vi "gxml_RcrsvFlatten.vi"(5 "Encap'd by Array?":bool, 6 "HierarchyInfo":T1, 7 "FlattenedData":string, 8 "error in":errorcluster, 9 "offset (0)":i32, 10 "Variant":variant, 11 "XML String In":string) -> (0 "error out":errorcluster, 1 "offset out":i32, 3 "XML String Out":string)   [LabVIEW 2011, in "Third Party VIs.lvlib" / "GXML.lvlib"]
doc: "This recursive VI is the core engine responsible for converting the LabVIEW cluster into an XML string. \n\nThe VI identifies the top level datatype of the input variant and recursively calls itself when an encapsulaing datatype is found (ie cluster or array). When a fundamental item is found (integer, boolean, etc) it is converted to text and given tags with appropriate attributes and hierarchy."
uses:
  GXML.lvlib
  <vilib>/Utility/VariantDataType/VariantType.lvlib
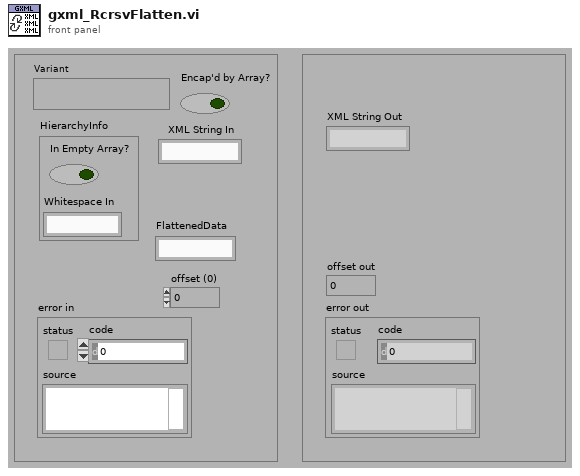
[diagram p1: front panel]
types:
  T1 = cluster{"In Empty Array?":bool, "Whitespace In":string}
  T2 = typedef "VariantType.lvlib/Type.ctl" = enum8{"Invalid Type", "Void", "I8", "I16", "I32", "I64", "U8", "U16", "U32", "U64", "Single Float", "Double Float", "Extended Float", "Single Complex", "Double Complex", "Extended Complex", "Enum U8", "Enum U16", "Enum U32", "Enum U64", "Single Float With Unit", "Double Float With Unit", "Extended Float With Unit", "Single Complex with Unit", "Double Complex with Unit", "Extended Complex with Unit", "Boolean", "String", "Path", "Picture", "Tag", "Array", "Cluster", "Variant", "LV Variant", "Waveform", "Timestamp", "Digital Waveform", "Digital Data", "ExpressData", "Refnum", "External Data", "VI", "Poly VI", "LabVIEW Class Instance", "Fixed Point"}
  T3 = cluster{"TypeAttr":string, "EnumSelAttr":string, "DataString":string}
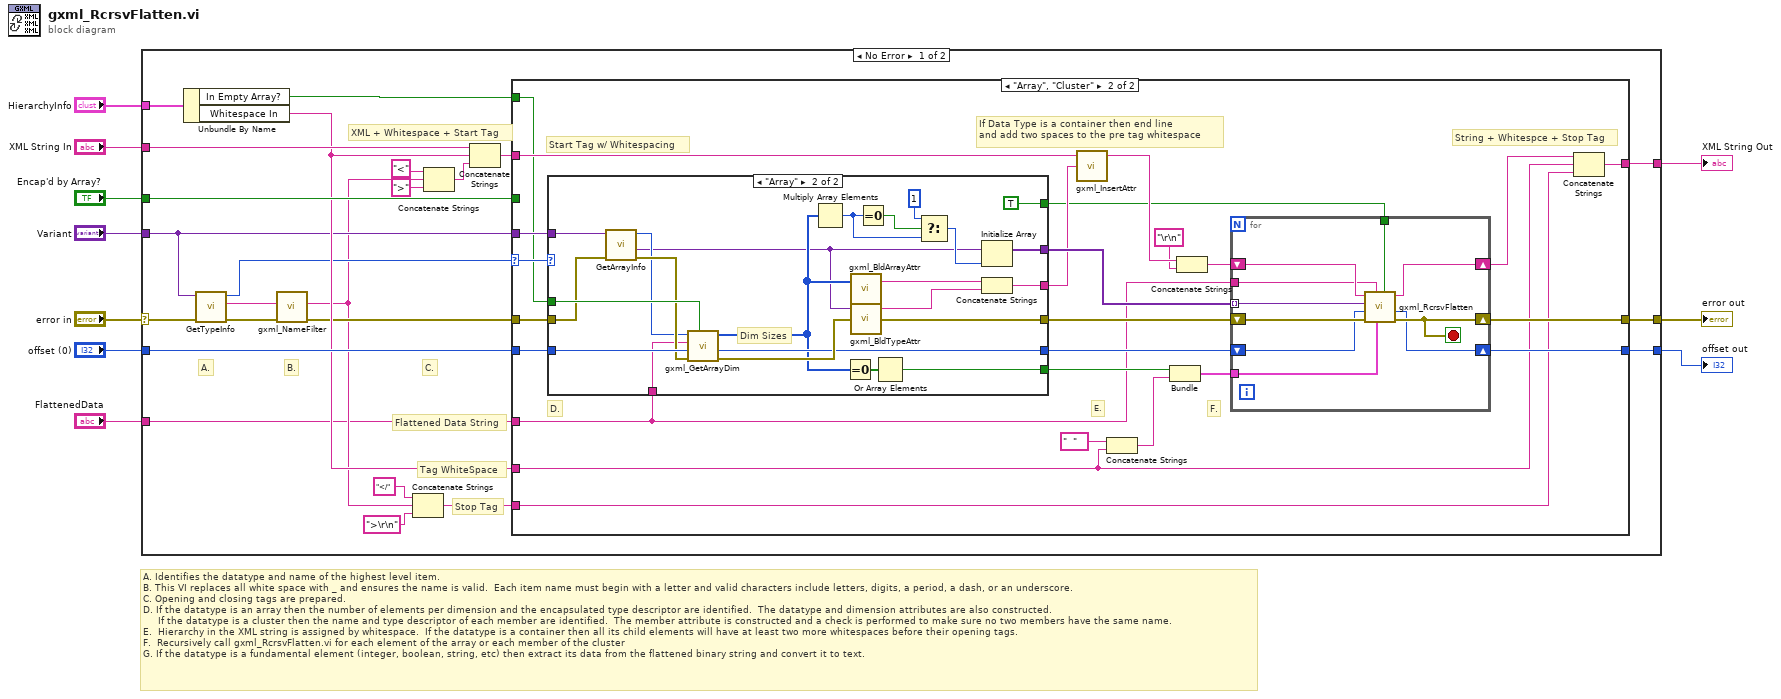
[diagram p0: block diagram]
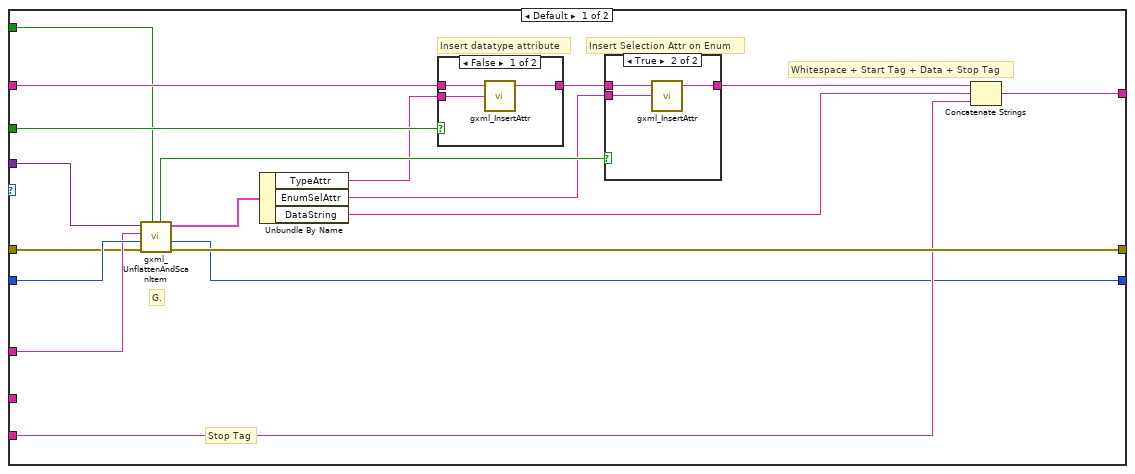
[diagram p2: hidden frame]
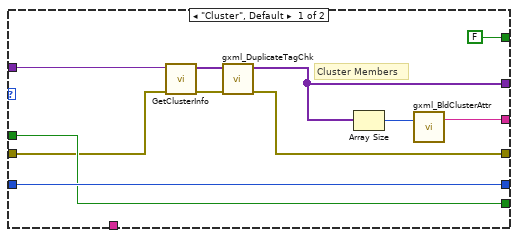
[diagram p5: hidden frame]
diagram:
  # "A. Identifies the datatype and name of the highest level item.\nB. This VI replaces all white space with _ and ensures the name is valid.  Each item name must begin with a letter and valid characters include letters, digits, a period, a dash, or an underscore.\nC. Opening and closing tags are prepared.\nD. If the datatype is an array then the number of elements per dimension and the encapsulated type descriptor are identified.  The datatype and dimension attributes are also constructed.\n     If the datatype is a cluster then the name and type descriptor of each member are identified.  The member attribute is constructed and a check is performed to make sure no two members have the same name.\nE.  Hierarchy in the XML string is assigned by whitespace.  If the datatype is a container then all its child elements will have at least two more whitespaces before their opening tags.\nF.  Recursively call gxml_RcrsvFlatten.vi for each element of the array or each member of the cluster\nG. If the datatype is a fundamental element (integer, boolean, string, etc) then extract its data from the flattened binary string and convert it to text."
  n1 = case shown="No Error" "error in" {
    selector: "error in" -> [w24 w132]
    tunnel: [w34 w132] -> w10
    tunnel: [w32 w131] -> w7
    tunnel: [w33 w130] -> w3
    tunnel: "XML String In" -> [w31 w131]
    tunnel: "Encap'd by Array?" -> [w29 _]
    tunnel: "HierarchyInfo" -> [w28 _]
    tunnel: "offset (0)" -> [w26 w130]
    tunnel: "Variant" -> [w22 _]
    tunnel: "FlattenedData" -> [w11 _]
    frame No Error {
      # "C."
      # "B."
      # "A."
      # "Flattened Data String"
      # "Stop Tag"
      # "XML + Whitespace + Start Tag"
      # "Tag WhiteSpace"
      n2 = Unbundle By Name(w28) -> ("In Empty Array?"=w27:bool, "Whitespace In"=w25:string)
      n3 = call <vilib>:"GetTypeInfo.vi"("error in (no error)"=w24, "Variant"=w22) -> ("error out"=w15:errorcluster, "Name"=w14:string, "Type Enum"=w23:T2)  [unwired: 5 in, 2 out]
      n4 = call "gxml_NameFilter.vi"("error in"=w15, "Tag Name"=w14) -> ("error out"=w13:errorcluster, "Tag_Name"=w12:string)  [unwired: 7 in]
      n5 = Concatenate Strings("</", w12, ">\r\n" ("string")) -> (w16:string)
      n6 = Concatenate Strings("<", w12, ">" ("string")) -> (w17:string)
      n7 = Concatenate Strings(w31, w25, w17) -> (w30:string)
      n8 = case shown="\"Array\", \"Cluster\"" w23 {
        selector: w23 -> [_ w80]
        tunnel: w22 -> [w39 w85]
        tunnel: w13 -> [w40 w84]
        tunnel: [w50 w74] -> w32
        tunnel: w26 -> [w52 w83]
        tunnel: [w51 w79] -> w34
        tunnel: [w42 w78] -> w33
        tunnel: w25 -> [_ w63]
        tunnel: w30 -> [w48 w72]
        tunnel: w16 -> [w49 w73]
        tunnel: w29 -> [w44 _]
        tunnel: w27 -> [w43 w68]
        tunnel: w11 -> [w41 w61]
        frame Default {
          # "G."
          # "Insert datatype attribute"
          # "Insert Selection Attr on Enum"
          # "Whitespace + Start Tag + Data + Stop Tag"
          # "Stop Tag"
          n9 = call "gxml_UnflattenAndScanItem.vi"("Disable Parse?"=w43, "error in"=w40, "Offset In"=w52, "FlattenedData"=w41, "variant"=w39) -> ("error out"=w51:errorcluster, "Offset Out"=w42:i32, "Data Info"=w38:T3, "Enum?"=w45:bool)  [unwired: 3 in]
          n10 = Unbundle By Name(w38) -> ("TypeAttr"=w37:string, "EnumSelAttr"=w36:string, "DataString"=w35:string)
          n11 = case shown="False" w44 {
            tunnel: w48 -> [w59 w60]
            tunnel: [w58 w60] -> w47
            tunnel: w37 -> [w57 _]
            frame False {
              n12 = call "gxml_InsertAttr.vi"("Attribute"=w57, "Input String"=w59) -> ("Output String"=w58:string)  [unwired: 3 in]
            }
            frame True {
            }
          }
          n13 = case shown="True" w45 {
            tunnel: w47 -> [w53 w56]
            tunnel: [w53 w55] -> w46
            tunnel: w36 -> [_ w54]
            frame False {
            }
            frame True {
              n14 = call "gxml_InsertAttr.vi"("Attribute"=w54, "Input String"=w56) -> ("Output String"=w55:string)  [unwired: 3 in]
            }
          }
          n15 = Concatenate Strings(w46, w35, w49) -> (w50:string)
        }
        frame "Array", "Cluster" {
          # "E."
          # "F."
          # "D."
          # "Start Tag w/ Whitespacing"
          # "If Data Type is a container then end line\nand add two spaces to the pre tag whitespace"
          # "String + Whitespce + Stop Tag"
          n16 = case shown="\"Array\"" w80 {
            tunnel: w85 -> [w90 w101]
            tunnel: w84 -> [w91 w103]
            tunnel: w83 -> [w93 w108]
            tunnel: [w87 w119] -> w82
            tunnel: [w86 w114] -> w81
            tunnel: [w95 w116] -> w70
            tunnel: [FALSE TRUE] -> w69
            tunnel: w68 -> [w92 w106]
            tunnel: [w93 w104] -> w67
            tunnel: [w92 w105] -> w66
            tunnel: w61 -> [_ w97]
            frame "Cluster", Default {
              # "Cluster Members"
              n17 = call <vilib>:"GetClusterInfo.vi"("error in (no error)"=w91, "Variant"=w90) -> ("error out"=w88:errorcluster, "Cluster Elements"=w89:variant[])  [unwired: 8 in]
              n18 = call "gxml_DuplicateTagChk.vi"("error in"=w88, "Cluster Elements"=w89) -> ("error out"=w86:errorcluster, "Cluster Elements Out"=w87:variant[])  [unwired: 7 in]
              n19 = Array Size(array=w87) -> (size(s)=w96:i32)
              n20 = call "gxml_BldClusterAttr.vi"("Num of Elements"=w96) -> ("ClusterAttrString"=w95:string)  [unwired: 2 in]
            }
            frame "Array" {
              # "Dim Sizes"
              n21 = call <vilib>:"GetArrayInfo.vi"("error in (no error)"=w103, "Variant"=w101) -> ("error out"=w102:errorcluster, "ArrayElement"=w98:variant, "NDims"=w100:i32)  [unwired: 6 in, 1 out]
              n22 = call "gxml_GetArrayDim.vi"("Empty Default Array?"=w106, "error in"=w102, "offset (0)"=w108, "Flattened Data String"=w97, "Dimensions"=w100) -> ("error out"=w115:errorcluster, "offset"=w104:i32, "ArrayDimensions"=w99:i32[])  [unwired: 3 in, 1 out]
              n23 = Multiply Array Elements(1:w99) -> (0:w112:i32)
              n24 = Equal To 0?(x=w99) -> (x = 0?=w107:bool[])
              n25 = call "gxml_BldArrayAttr.vi"("Dim Sizes"=w99) -> ("Dim Attr String"=w118:string)  [unwired: 2 in]
              n26 = call "gxml_BldTypeAttr.vi"("error out"=w115, "Variant"=w98) -> ("error IO"=w114:errorcluster, "TypeString"=w117:string)  [unwired: 2 in]
              n27 = Equal To 0?(x=w112) -> (x = 0?=w113:bool)
              n28 = Or Array Elements(Boolean array=w107) -> (logical OR=w105:bool)
              n29 = Select(t=1, s=w113, f=w112) -> (s? t:f=w110:i32)
              n30 = Initialize Array(w98, w110) -> (w119:variant[])
              n31 = Concatenate Strings(w118, w117) -> (w116:string)
            }
          }
          n32 = call "gxml_InsertAttr.vi"("Attribute"=w70, "Input String"=w72) -> ("Output String"=w71:string)  [unwired: 3 in]
          n33 = Concatenate Strings("  " ("string"), w63) -> (w62:string)
          n34 = Bundle("In Empty Array?"=w66, w62) -> (w65:cluster{"In Empty Array?":bool, string})  [unwired: 1 in]
          n35 = Concatenate Strings(w71, "\r\n" ("string")) -> (w76:string)
          n36 = for {
            shift-right: [w129] -> w75
            shift-left: w76 -> [w127]
            shift-right: [w123] -> w78
            shift-left: w67 -> [w124]
            tunnel: w82 -> [w121] mode=indexing
            tunnel: w69 -> [w125]
            tunnel: w65 -> [w122]
            shift-right: [w126] -> w79
            shift-left: w81 -> [w128]
            tunnel: w61 -> [w120]
            stop <- w126 stop-if-true
            n37 = call "gxml_RcrsvFlatten.vi"("Encap'd by Array?"=w125, "HierarchyInfo"=w122, "FlattenedData"=w120, "error in"=w128, "offset (0)"=w124, "Variant"=w121, "XML String In"=w127) -> ("error out"=w126:errorcluster, "offset out"=w123:i32, "XML String Out"=w129:string)  [unwired: 2 in]
          }
          n38 = Concatenate Strings(w75, w63, w73) -> (w74:string)
        }
      }
    }
    frame Error {
    }
  }
  "error out" <- w10
  "XML String Out" <- w7
  "offset out" <- w3
